vi "swmm_open.vi"(3 "Display success msg":bool, 5 "SWMM Input File (.inp)":path) -> (0 "error out":errorcluster)   [LabVIEW 2014]
uses:
  swmm5.dll
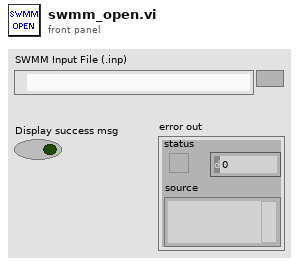
[diagram p1: front panel]
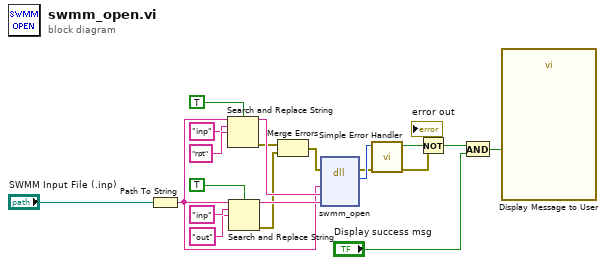
[diagram p0: block diagram]
diagram:
  n1 = Path To String(path="SWMM Input File (.inp)") -> (string=w12:string)
  n2 = Search and Replace String(case sensitive?=TRUE ("ignore case? (F)"), input string=w12, search string="inp" ("substring (\"\")"), replace string="rpt" ("replace string (\"\")")) -> (result string=w14:string, error out=w8:errorcluster)  [unwired: 4 in, 2 out]
  n3 = Search and Replace String(case sensitive?=TRUE ("ignore case? (F)"), input string=w12, search string="inp" ("substring (\"\")"), replace string="out" ("replace string (\"\")")) -> (result string=w13:string, error out=w7:errorcluster)  [unwired: 4 in, 2 out]
  n4 = Merge Errors(w8, w7) -> (w6:errorcluster)
  n5 = dll-call lib="PTH2zabs CUsers\nandres riañoDropboxProyecto AguasSoftwareMatSWMMMatSWMM 5.1.009LabVIEW modulex64\tswmm5.dll" fn="swmm_open"(error in=w6, "input"=w12, "report"=w14, "output"=w13) -> (error out=w9:errorcluster, "return type"=w10:i32)  [unwired: 5 in, 1 out]
  n6 = call <vilib>:"Simple Error Handler.vi"("error code (no error:0)"=w10, "error in (no error)"=w9) -> ("error?"=w5:bool, "error out"=→"error out":errorcluster)  [unwired: 3 in, 3 out]
  n7 = Not(x=w5) -> (.not. x?=w4:bool)
  n8 = And(x=w4, y="Display success msg") -> (x .and. y?=w2:bool)
  n9 = call "Display Message to User"("Enable"=w2) -> ()  [unwired: 9 in, 2 out]
